vi "topology file to cluster.vi"(8 "error in (no error)":errorcluster, 11 "Path":path) -> (0 "error out":errorcluster, 2 "topology":T1)   [LabVIEW 2015, in "SLSC Switch.lvclass"]
uses:
  SLSC Switch.lvclass
  Controls/JSON.Topology.ctl
  Controls/JSON.InitialState.ctl
  Controls/JSON.ChannelList.ctl
  Controls/JSON.ConnectionList.ctl
  <vilib>/Utility/config.llb/Read Key (String).vi
  <vilib>/Utility/config.llb/NI_LVConfig.lvlib
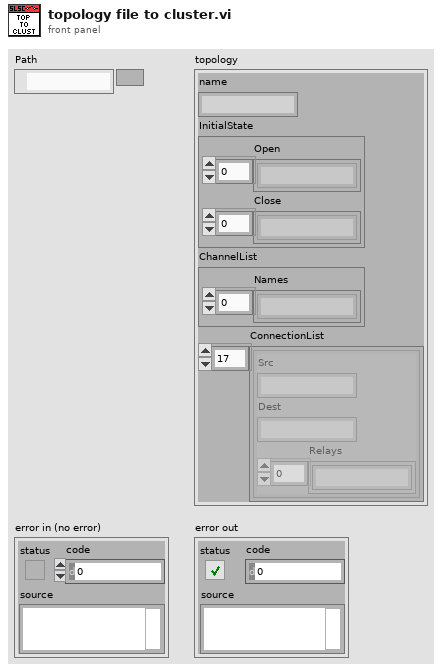
[diagram p1: front panel]
types:
  T1 = typedef "SLSC Switch.lvclass/JSON.Topology.ctl" = cluster{"name":string, "InitialState":T2, "ChannelList":T3, "ConnectionList":T4[]}
  T2 = typedef "SLSC Switch.lvclass/JSON.InitialState.ctl" = cluster{"Open":string[], "Close":string[]}
  T3 = typedef "SLSC Switch.lvclass/JSON.ChannelList.ctl" = cluster{"Names":string[]}
  T4 = typedef "SLSC Switch.lvclass/JSON.ConnectionList.ctl" = cluster{"Src":string, "Dest":string, "Relays":string[]}
  T5 = typedef "NI_LVConfig.lvlib/Config Data RefNum.ctl" = refnum<k1>
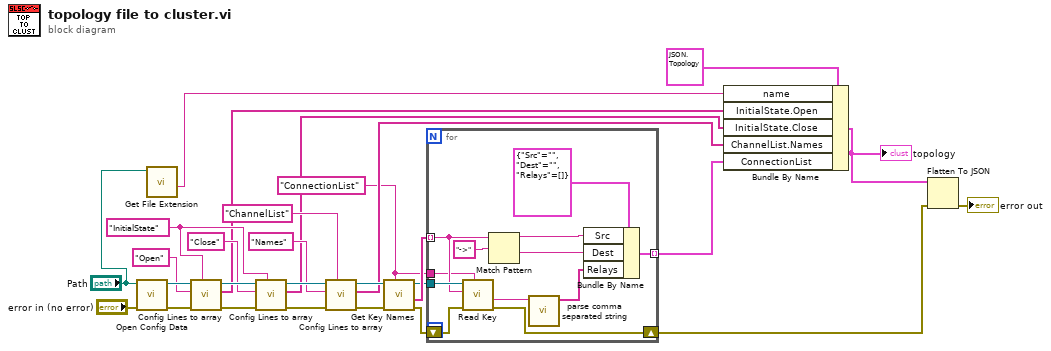
[diagram p0: block diagram]
diagram:
  w7 = "ConnectionList" ("section")
  w23 = "InitialState" ("section")
  n1 = call <vilib>:"Open Config Data.vi"("error in (no error)"="error in (no error)", "configuration file path"="Path") -> ("error out"=w28:errorcluster, "refnum"=w27:T5)  [unwired: 7 in, 1 out]
  n2 = call <vilib>:"Get File Extension.vi"("file"="Path") -> ("filename without extension"=w1:string)  [unwired: 6 in, 4 out]
  n3 = call "Config Lines to array.vi"("section"=w23, "error in (no error)"=w28, "Key Name"="Open" ("string"), "Refnum in"=w27) -> ("error out"=w25:errorcluster, "Array"=w14:string[], "Refnum out"=w26:T5)  [unwired: 5 in]
  n4 = call "Config Lines to array.vi"("section"=w23, "error in (no error)"=w25, "Key Name"="Close", "Refnum in"=w26) -> ("error out"=w20:errorcluster, "Array"=w13:string[], "Refnum out"=w21:T5)  [unwired: 5 in]
  n5 = call "Config Lines to array.vi"("section"="ChannelList", "error in (no error)"=w20, "Key Name"="Names", "Refnum in"=w21) -> ("error out"=w16:errorcluster, "Array"=w12:string[], "Refnum out"=w17:T5)  [unwired: 5 in]
  n6 = call <vilib>:"Get Key Names.vi"("section"=w7, "error in (no error)"=w16, "refnum"=w17) -> ("error out"=w8:errorcluster, "key names"=w11:string[], "refnum out"=w10:T5)  [unwired: 5 in, 1 out]
  n7 = for {
    tunnel: w11 -> [w36] mode=indexing
    tunnel: w10 -> [w39]
    tunnel: [w32] -> w9 mode=indexing
    tunnel: w7 -> [w30]
    shift-right: [w29] -> w5
    shift-left: w8 -> [w31]
    n8 = call-poly <vilib>:"Read Key.vi"("section"=w30, "error in (no error)"=w31, "key"=w36, "refnum"=w39) -> ("error out"=w29:errorcluster, "value"=w38:string)  [unwired: 4 in, 2 out]
    n9 = Match Pattern(string=w36, regular expression="->") -> (before substring=w34:string, after substring=w33:string)  [unwired: 1 in, 2 out]
    n10 = call "parse comma separated string.vi"("String"=w38) -> ("Array"=w37:string[])  [unwired: 10 in]
    n11 = Bundle By Name(cluster=T4 {"Src"="", "Dest"="", "Relays"=[]} ("ConnectionList"), "Src"=w34, "Dest"=w33, "Relays"=w37) -> (w32:T4)
  }
  n12 = Bundle By Name(cluster=T1 {"name"="", "InitialState"={"Open"=["k0", "k1", "k2", "k3", "k4", "k5"], "Close"=[]}, "ChannelList"={"Names"=["a", "b", "c", "d", "e", "f", "g"]}, "ConnectionList"=[{"Src"="a", "Dest"="b", "Relays"=["k0"]}, {"Src"="b", "Dest"="c", "Relays"=["k1"]}, {"Src"="c", "Dest"="d", "Relays"=["k2"]}]} ("Topology"), "name"=w1, "InitialState.Open"=w14, "InitialState.Close"=w13, "ChannelList.Names"=w12, "ConnectionList"=w9) -> (w6:T1)
  "topology" <- w6
  n13 = Flatten To JSON(anything=w6, error in (no error)=w5) -> (11:→"error out":errorcluster)  [unwired: 1 in, 1 out]
